vi "LifetimeHistograms.vi"(1 "input lifetime histograms":T1 {"channel width (ns)" format="%.2f"}, 2 "set":bool) -> (0 "output lifetime histograms":T1 {"channel width (ns)" format="%.2f"})   [LabVIEW 2009]
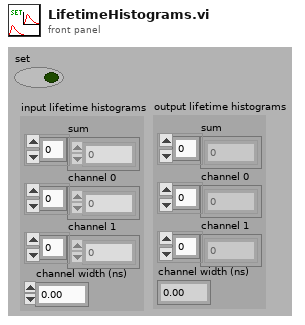
[diagram p1: front panel]
types:
  T1 = cluster{"sum":u32[], "channel 0":u32[], "channel 1":u32[], "channel width (ns)":dbl}
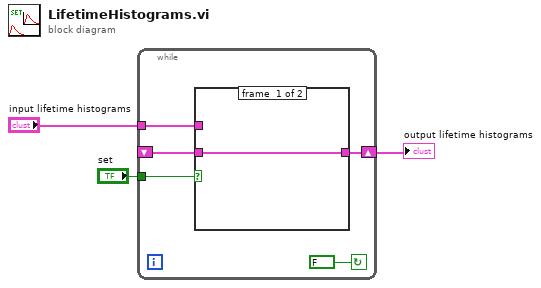
[diagram p0: block diagram]
diagram:
  n1 = while {
    shift-right: [w6] -> w2
    shift-left: _ -> [w4]
    tunnel: "set" -> [w7]
    tunnel: "input lifetime histograms" -> [w5]
    stop <- FALSE continue-if-true
    n2 = case shown="True" w7 {
      tunnel: [w9 w10] -> w6
      tunnel: w5 -> [_ w10]
      tunnel: w4 -> [w9 _]
      frame #0 {
      }
      frame #1 {
      }
    }
  }
  "output lifetime histograms" <- w2
